vi "Y Axis Acceleration Conversion sub_VI.vi"(2 "Deceleration (mm/s^2)":dbl, 3 "Acceleration (mm/s^2)":dbl) -> (0 "Freq decrease per 0.1ms (Hz)":dbl, 1 "Freq increase per 0.1ms (Hz)":dbl)   [LabVIEW 2017]
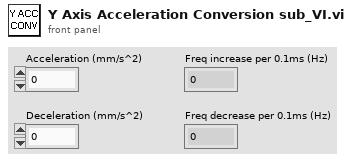
[diagram p1: front panel]
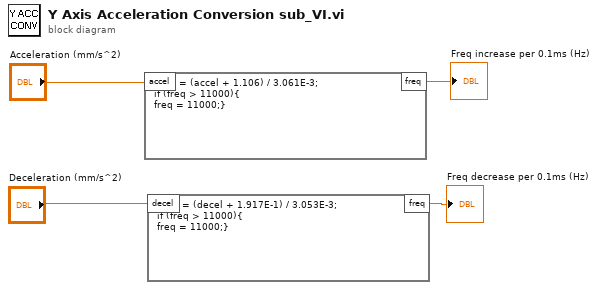
[diagram p0: block diagram]
diagram:
  n1 = formula code="freq  = (accel + 1.106) / 3.061E-3;\nif (freq > 11000){\nfreq = 11000;}"("accel"="Acceleration (mm/s^2)") -> ("freq"=→"Freq increase per 0.1ms (Hz)":dbl)
  n2 = formula code="freq  = (decel + 1.917E-1) / 3.053E-3;\nif (freq > 11000){\nfreq = 11000;}"("decel"="Deceleration (mm/s^2)") -> ("freq"=→"Freq decrease per 0.1ms (Hz)":dbl)
